vi "DIO_Write1.vi"(7 "Device Index":u32 max=32, 8 "error in (no error)":errorcluster, 10 "Data":bool, 11 "Bit Index":u32) -> (0 "error out":errorcluster)   [LabVIEW 2012]
doc: "This VI can be used to write a single bit on an ACCES USB-DIO board."
uses:
  Windows/System32/AIOUSB.dll
panel:
  out "Return Value":u32
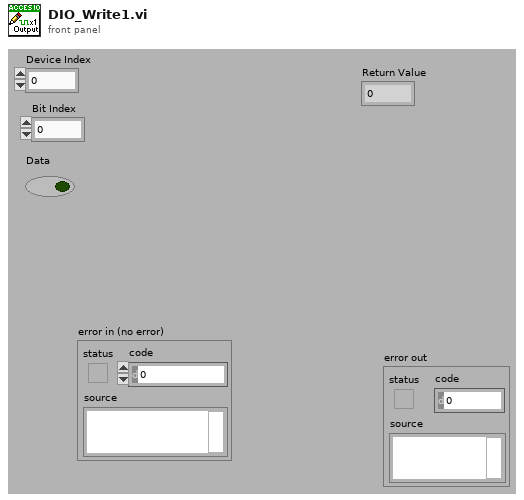
[diagram p1: front panel]
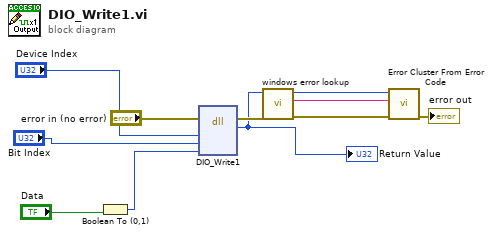
[diagram p0: block diagram]
diagram:
  n1 = Boolean To (0,1)(Boolean="Data") -> (0, 1=w9:i16)
  n2 = dll-call lib="C:/Windows/System32/AIOUSB.dll" fn="DIO_Write1"(error in="error in (no error)", "DeviceIndex"="Device Index", "BitIndex"="Bit Index", "bData"=w9) -> (error out=w3:errorcluster, w1:u32)  [unwired: 5 in, 1 out]
  "Return Value" <- w1
  n3 = call "windows error lookup.vi"("error in (no error)"=w3, "Error Code"=w1) -> ("error out"=w4:errorcluster, "error message (\"\")"=w6:string)  [unwired: 8 in]
  n4 = call <vilib>:"Error Cluster From Error Code.vi"("error in (no error)"=w4, "error message (\"\")"=w6, "error code (0)"=w1) -> ("error out"=→"error out":errorcluster)  [unwired: 6 in]
